vi "PH_Cont-601k_PowerUnit.scr Set READY.vi"(0 "VI in":refnum<vi>, 5 "error in (no error)":errorcluster) -> (14 "VI out":refnum<vi>, 19 "error out":errorcluster)   [LabVIEW 2014, in "PH_Cont-601k_PowerUnit.lvlib"]
uses:
  PH_Cont-601k_PowerUnit.lvlib
  PH_Basics/PH_PowerUnit_BaseClass/PH_PowerUnit_BaseClass.SM States.ctl
  PH_Basics/PH_PowerUnit_BaseClass/PH_PowerUnit_BaseClass.lvlib
  PH_Devices/PH_Cont-601k_PSU/PH_Cont-601k_PSU.lvlib
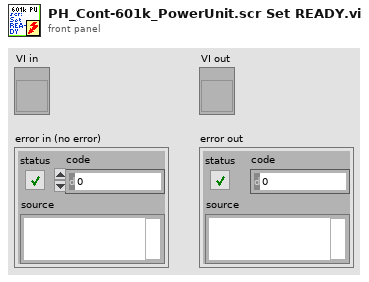
[diagram p1: front panel]
types:
  T1 = typedef "PH_PowerUnit_BaseClass.lvlib/PH_PowerUnit_BaseClass.SM States.ctl" = enum16{".", "Stand by", "Switch PU on", "Configure", "Set Default Voltage", "Set STANDBY", "Set READY", "Wait for Shot Cmd", "Open Dump Rods", "Open Ross Relais", "Close Ross Relais", "Switch PSU on", "Switch PSU off", "Charge", "Switch GD Channel on", "Close Dump Rods", "Rods-TO", "RR-TO", "PSU-TO", "Trigger-TO"}
  T2 = typedef "PH_Cont-601k_PSU.lvlib/PH_Cont-601k_PSU.i attribute.ctl" = cluster{"GUI Refs":T3, "Interlock":bool, "Service ID applied Voltage":i32, "Device Settings":cluster{"Configuration":T4, "Flash Interval [s]":dbl, "Mode":T5, "Voltage [V]":u16, "Charge":bool, "VISA resource name":refnum<visa-resource-name>}, "Readyness":T6, "Information":cluster{"VISA resource name":refnum<visa-resource-name>, "Tagname Power On":string, "Interlock":cluster{"Instance":string, "Tagname":string}, "Limits [V]":cluster{"Lower":dbl, "Upper":dbl}, "Tagname PSU On":string}, "R2S":bool, "Charge is allowed":bool}
  T3 = typedef "PH_Cont-601k_PSU.lvlib/PH_Cont-601k_PSU.GUI Refs.ctl" = cluster{"Power On":refnum<vi>, "Hard- and Software":refnum<vi>, "Device Status":refnum<vi>, "Device Error":refnum<vi>, "Configuration":refnum<vi>, "Flash Interval [s]":refnum<vi>, "Interlock":refnum<vi>, "Interlock Indicator":refnum<vi>, "Voltage [V]":refnum<vi>, "Readyness":refnum<vi>, "Mode":refnum<vi>, "Reset Error":refnum<vi>, "Expert working":refnum<vi>, "Charge":refnum<vi>, "PSU On":refnum<vi>}
  T4 = typedef "PH_Cont-601k_PSU.lvlib/PH_Cont-601k_PSU.Configuration.ctl" = u16
  T5 = typedef "PH_Cont-601k_PSU.lvlib/PH_Cont-601k_PSU.Mode.ctl" = enum32{"STOP", "STANDBY", "READY", "EMISSION", "ERROR"}
  T6 = typedef "PH_Cont-601k_PSU.lvlib/PH_Cont-601k_PSU.Readyness.ctl" = cluster{"Program":T7, "Device":T8}
  T7 = typedef "PH_Cont-601k_PSU.lvlib/PH_Cont-601k_PSU.Readyness Program.ctl" = enum32{"OFF", "POWER", "INTERLOCK"}
  T8 = typedef "PH_Cont-601k_PSU.lvlib/PH_Cont-601k_PSU.Readyness Device.ctl" = enum32{"OFF", "CONNECTING", "CONNECTED", "OPERATING", "EOC", "ERROR"}
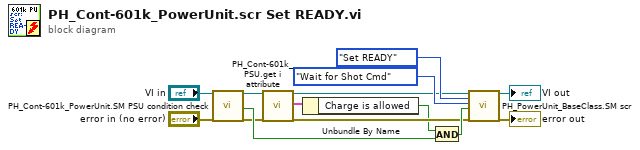
[diagram p0: block diagram]
diagram:
  n1 = call "PH_Cont-601k_PowerUnit.SM PSU condition check.vi"("VI in"="VI in", "error in (no error)"="error in (no error)") -> ("VI out"=w6:refnum<vi>, "Condition fullfilled"=w8:bool, "error out"=w5:errorcluster)  [unwired: 15 in]
  n2 = call "PH_Cont-601k_PSU.get i attribute.vi"("i ref in"=w6, "error in (no error)"=w5) -> ("i ref out"=w4:refnum<vi>, "i attribute"=w2:T2, "error out"=w3:errorcluster)  [unwired: 15 in]
  n3 = Unbundle By Name(w2) -> ("Charge is allowed"=w1:bool)
  n4 = And(x=w1, y=w8) -> (x .and. y?=w7:bool)
  n5 = call "PH_PowerUnit_BaseClass.SM scr.vi"("VI in"=w4, "Current SM State (condition)"=PH_PowerUnit_BaseClass.SM_States."Set READY", "Wanted SM State"=PH_PowerUnit_BaseClass.SM_States."Wait for Shot Cmd", "Further change condition"=w7, "error in (no error)"=w3) -> ("VI out"=→"VI out":refnum<vi>, "error out"=→"error out":errorcluster)  [unwired: 13 in]
